vi "DenoiseFIlter.vi"(1 "Filter Level":i32, 2 "Singal Input":i16) -> (0 "Signal Output":i16)   [LabVIEW 2020]
panel:
  out "Post-Filter":i16(graph)
  out "Pre-Filter":i16(graph)
  # "Leave these as is, they are for the wire input and output for\nthe sub-vi"
  # "Change this to be the number of points that you want to check\nfor the filter"
  # "Two charts for a sid-by-side comparison to make sure that the signal is being filtered enough"
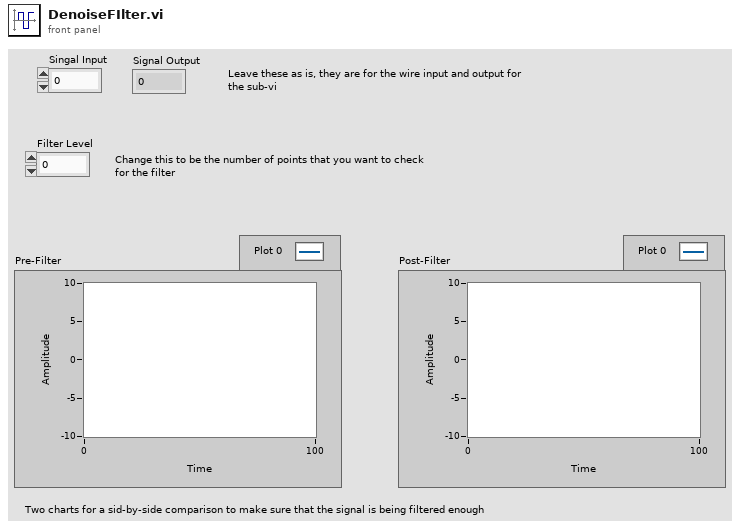
[diagram p1: front panel]
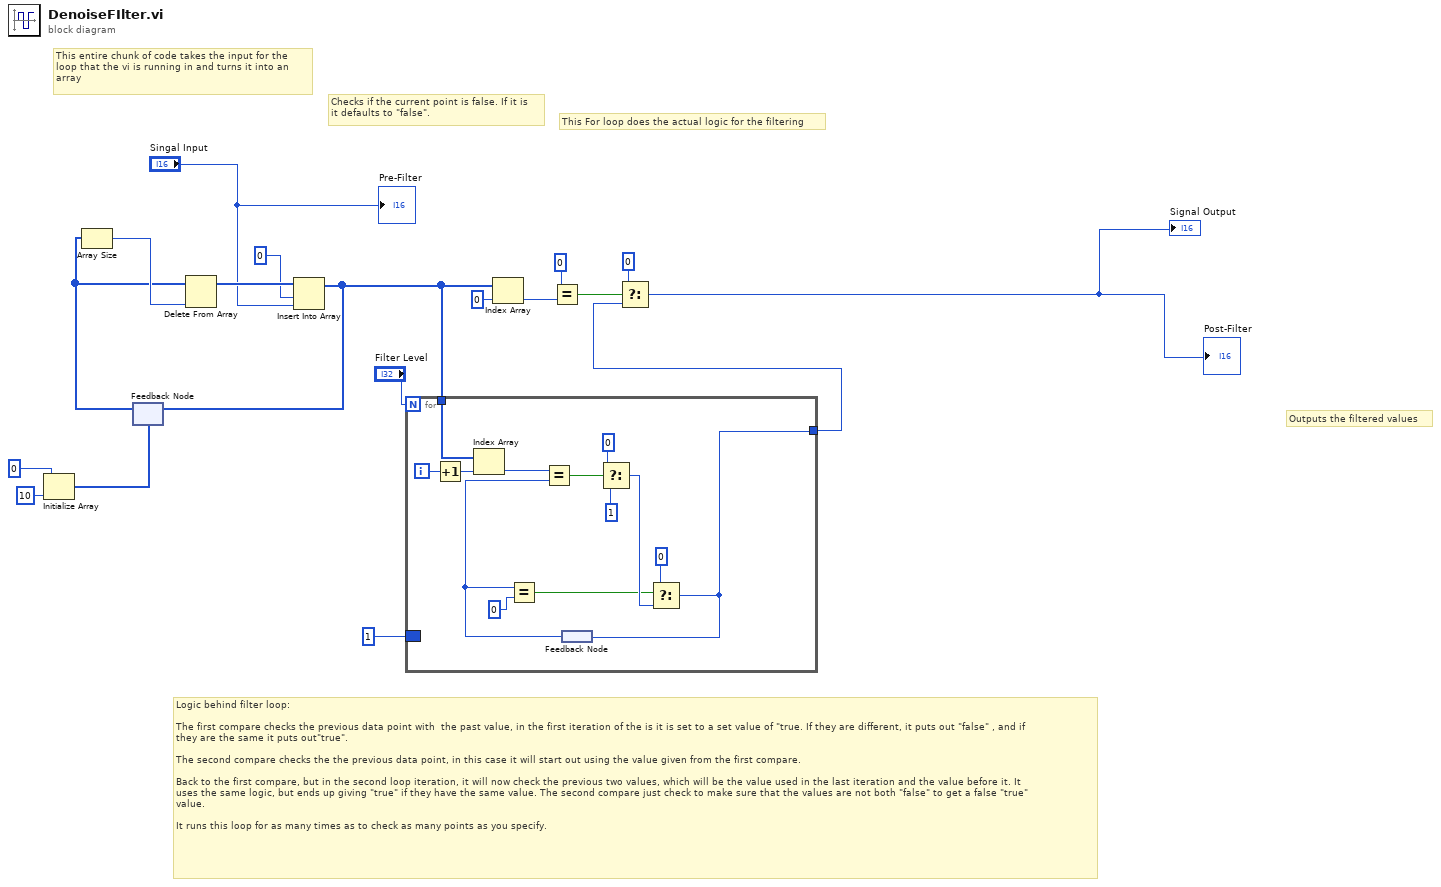
[diagram p0: block diagram]
diagram:
  # "Logic behind filter loop:\n\nThe first compare checks the previous data point with  the past value, in the first iteration of the is it is set to a set value of \"true. If they are different, it puts out \"false\" , and if \nthey are the same it puts out\"true\".\n\nThe second compare checks the the previous data point, in this case it will start out using the value given from the first compare.\n\nBack to the first compare, but in the second loop iteration, it will now check the previous two values, which will be the value used in the last iteration and the value before it. It \nuses the same logic, but ends up giving \"true\" if they have the same value. The second compare just check to make sure that the values are not both \"false\" to get a false \"true\"\nvalue.\n\nIt runs this loop for as many times as to check as many points as you specify."
  # "Checks if the current point is false. If it is\nit defaults to \"false\"."
  # "Outputs the filtered values"
  # "This entire chunk of code takes the input for the\nloop that the vi is running in and turns it into an \narray"
  # "This For loop does the actual logic for the filtering"
  n1 = Initialize Array(i16 0 ("element"), 10 ("dimension size")) -> (w18:i16[])
  n2 = feedback #1(w18) -> (w14:i16[])
  n3 = Array Size(array=w14) -> (size(s)=w15:i32)
  n4 = Delete From Array(array=w14, index=w15) -> (array with subset deleted=w13:i16[])  [unwired: 1 in, 1 out]
  n5 = Insert Into Array(array=w13, index=0, new element="Singal Input") -> (w5:i16[])
  n6 = feedback-in #1(w5) -> ()
  n7 = for {
    N: "Filter Level" -> [_]
    tunnel: w5 -> [w31]
    border: i16 1 -> [_]
    tunnel: [w23] -> w3
    i -> [w30]
    n8 = Increment(x=w30) -> (x+1=w29:i32)
    n9 = Index Array(array=w31, index=w29) -> (element=w28:i16)
    n10 = feedback #2() -> (w21:i16)
    n11 = Equal?(x=w21, y=i16 0) -> (x = y?=w19:bool)
    n12 = Equal?(x=w28, y=w21) -> (x = y?=w27:bool)
    n13 = Select(t=i16 0, s=w27, f=i16 1) -> (s? t:f=w22:i16)
    n14 = Select(t=i16 0, s=w19, f=w22) -> (s? t:f=w23:i16)
    n15 = feedback-in #2(w23) -> ()
  }
  n16 = Index Array(array=w5, index=0) -> (element=w10:i16)
  n17 = Equal?(x=i16 0, y=w10) -> (x = y?=w8:bool)
  n18 = Select(t=i16 0, s=w8, f=w3) -> (s? t:f=→"Signal Output" →"Post-Filter":i16)
  "Pre-Filter" <- "Singal Input"
